vi "Louver K.vi"(11 "Louver Position":dbl) -> (3 "K":dbl)   [LabVIEW 2019]
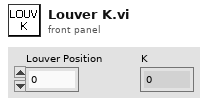
[diagram p1: front panel]
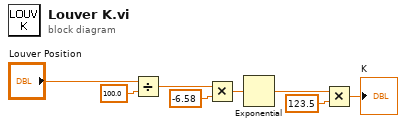
[diagram p0: block diagram]
diagram:
  n1 = Divide(x="Louver Position", y=100.0) -> (x/y=w7:dbl)
  n2 = Multiply(x=w7, y=-6.58) -> (x*y=w3:dbl)
  n3 = Exponential(1:w3) -> (0:w2:dbl)
  n4 = Multiply(x=w2, y=123.5) -> (x*y=→"K":dbl)
